vi "Database Drop Table.vi"(8 "error in (no error)":errorcluster, 10 "Table Name (\"\")":string, 11 "Connection Refnum":T1) -> (0 "error out":errorcluster, 3 "Connection Refnum":T1)   [LabVIEW 2011]
uses:
  SI.LIB/ODBC/SQL Controls/Connection Refnum.ctl
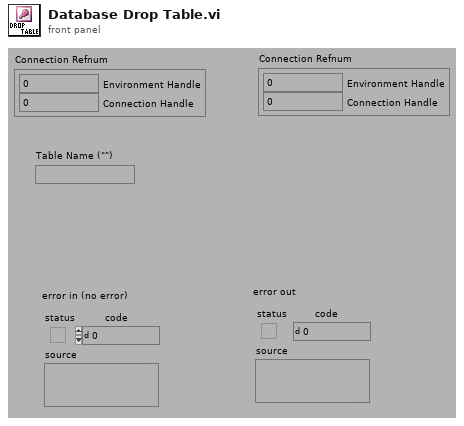
[diagram p1: front panel]
types:
  T1 = typedef "Connection Refnum.ctl" = cluster{"Environment Handle":i32, "Connection Handle":i32}
  T2 = typedef "Statement Refnum.ctl" = cluster{"Statement Handle":i32, "Parameter Number":u16}
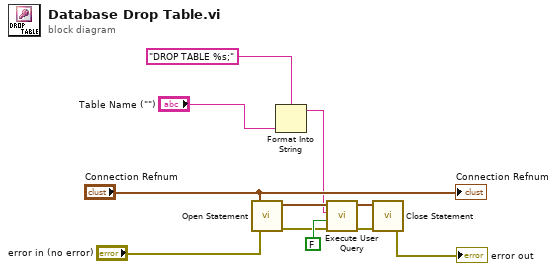
[diagram p0: block diagram]
diagram:
  n1 = call "Open Statement.vi"("error in (no error)"="error in (no error)", "Connection Refnum"="Connection Refnum") -> ("error out"=w9:errorcluster, "Statement Refnum"=w10:T2)  [unwired: 4 out]
  n2 = Format Into String(format string="DROP TABLE %s;" ("User Query"), "Table Name (\"\")") -> (resulting string=w2:string)  [unwired: 2 in, 1 out]
  n3 = call "Execute User Query.vi"("error in (no error)"=w9, "Return Data? (f)"=FALSE, "User Query"=w2, "Statement Refnum"=w10) -> ("error out"=w8:errorcluster, "Statement Refnum"=w7:T2)  [unwired: 2 out]
  n4 = call "Close Statement.vi"("error in (no error)"=w8, "Statement Refnum"=w7) -> ("error out"=→"error out":errorcluster)  [unwired: 5 out]
  "Connection Refnum" <- "Connection Refnum"
